vi "Memory.Pointer.U64.New.vi"(8 "error in (no error)":errorcluster) -> (0 "error out":errorcluster, 3 "U64 Pointer":refnum<class "Memory.Pointer.U64.lvclass">)   [LabVIEW 2016, in "Memory.Pointer.U64.lvclass"]
doc: "Allocates a new block of memory, represented by Pointer."
uses:
  Memory.Pointer.U64.lvclass
  Pointer.Numeric/Memory.Pointer.Numeric.lvclass
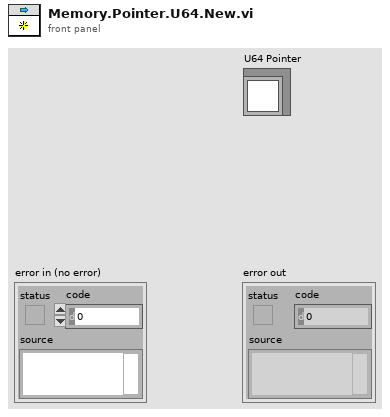
[diagram p1: front panel]
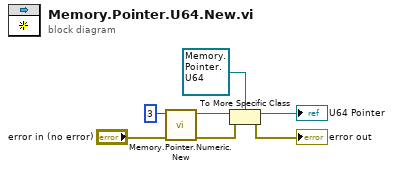
[diagram p0: block diagram]
diagram:
  n1 = call "Memory.Pointer.Numeric.New.vi"("error in (no error)"="error in (no error)", "power of 2"=i16 3) -> ("error out"=w5:errorcluster, "Numeric Pointer out"=w6:refnum<class "Memory.Pointer.Numeric.lvclass">)  [unwired: 8 in]
  n2 = To More Specific Class(target class=refnum<class "Memory.Pointer.U64.lvclass"> refnum ("LabVIEW Memory Manager.lvlib:DBL Pointer"), reference=w6, error in=w5) -> (specific class reference=→"U64 Pointer":refnum<class "Memory.Pointer.U64.lvclass">, error out=→"error out":errorcluster)
